vi "rs3_ExtractColor5.vi"(0 "Manual \nWhite Balance":bool, 1 "24bit Color Array":u8[](array[numeric])=array[921600 elements], 2 "AWB SW":bool, 3 "Alpha":dbl, 5 "Red":dbl=2.0, 6 "X offset":dbl, 7 "Color format":enum16{"Monochrome", "RGB internal (RGB)"}(ring), 9 "Green":dbl=1.0, 10 "Depth Y":i32=360, 11 "Blue":dbl=2.0, 12 "RGB  X":i32=640, 13 "Gain":dbl=2.0, 14 "RGB Y":i32=480, 15 "Depth X":i32=480) -> (4 "Norm Mesh Color":T1(array[cluster]))   [LabVIEW 2018, in "libRealSense3.lvlib"]
doc: "Extract the color in a format required for plotting a pointcloud into 3D picture indication"
uses:
  libRealSense3.lvlib
  <vilib>/Analysis/NI_AALBase.lvlib
panel:
  out "New Blue":dbl
  out "New Green":dbl
  out "New Red":dbl
  out "Ratio X":dbl=1.0
  out "Ratio Y":dbl=640.0
  # "RS3 Extract Color for PointCloud"
  # "(C) Intel Corp. 2017,  AGJ"
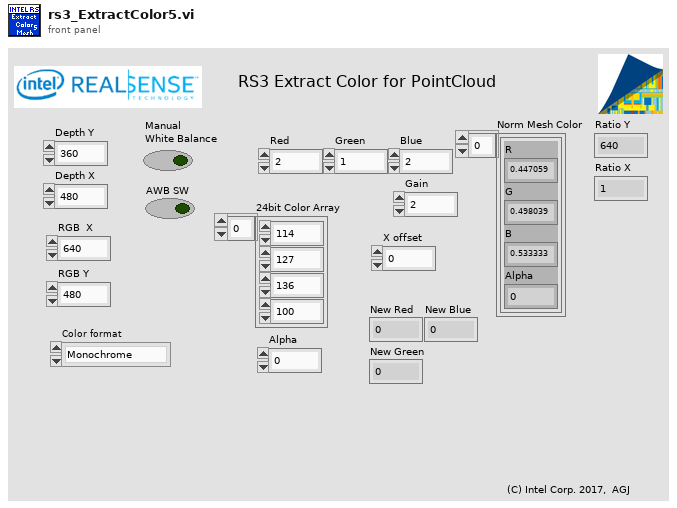
[diagram p1: front panel]
types:
  T1 = cluster{"R":dbl, "G":dbl, "B":dbl, "Alpha":dbl}[]
  T2 = cluster{"upper limit":dbl, "upper limit":dbl, "upper limit":dbl, u8}
  T3 = cluster{"upper limit":dbl, "upper limit":dbl, "upper limit":dbl, "Alpha":dbl}
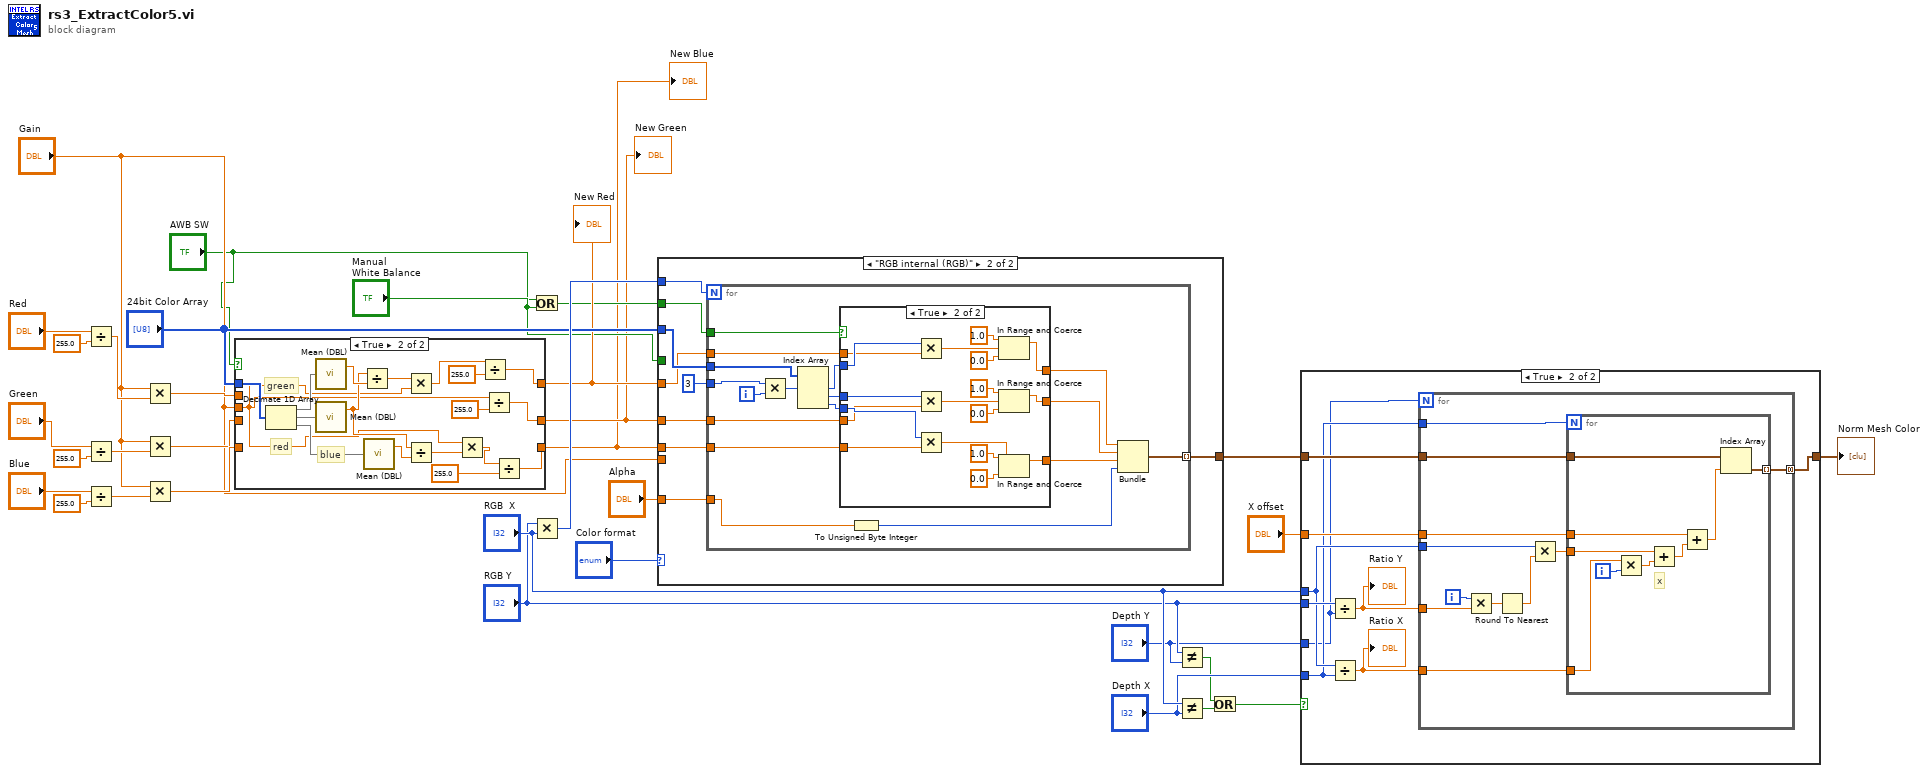
[diagram p0: block diagram]
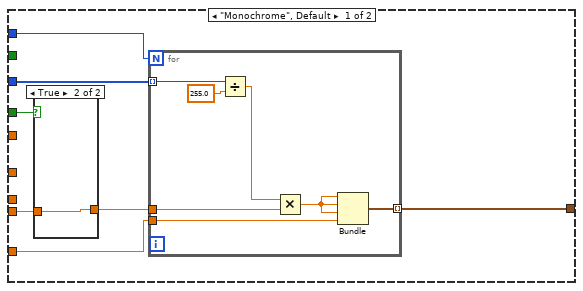
[diagram p3: hidden frame]
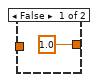
[diagram p4: hidden frame]
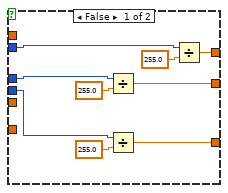
[diagram p5: hidden frame]
diagram:
  n1 = Divide(x="Red", y=255.0 ("upper limit")) -> (x/y=w13:dbl)
  n2 = Divide(x="Green", y=255.0 ("upper limit")) -> (x/y=w12:dbl)
  n3 = Divide(x="Blue", y=255.0 ("upper limit")) -> (x/y=w11:dbl)
  n4 = Multiply(x="Gain", y=w13) -> (x*y=w8:dbl)
  n5 = Multiply(x="Gain", y=w12) -> (x*y=w9:dbl)
  n6 = Multiply(x="Gain", y=w11) -> (x*y=w10:dbl)
  n7 = case shown="True" "AWB SW" {
    tunnel: "24bit Color Array" -> [_ w54]
    tunnel: [w34 w40] -> w14
    tunnel: [w36 w44] -> w2
    tunnel: w9 -> [w36 _]
    tunnel: w10 -> [w35 _]
    tunnel: [w35 w37] -> w1
    tunnel: w8 -> [w34 _]
    tunnel: "Gain" -> [_ w45]
    frame False {
    }
    frame True {
      # "blue"
      # "green"
      # "red"
      n8 = Decimate 1D Array(w54) -> (w53:u8[], w52:u8[], w51:u8[])
      n9 = call <vilib>:"Mean (DBL).vi"("X"=w53) -> ("mean"=w50:dbl)  [unwired: 1 out]
      n10 = call <vilib>:"Mean (DBL).vi"("X"=w52) -> ("mean"=w47:dbl)  [unwired: 1 out]
      n11 = Divide(x=w47, y=w50) -> (x/y=w48:dbl)
      n12 = call <vilib>:"Mean (DBL).vi"("X"=w51) -> ("mean"=w49:dbl)  [unwired: 1 out]
      n13 = Multiply(x=w48, y=w45) -> (x*y=w42:dbl)
      n14 = Divide(x=w47, y=w49) -> (x/y=w46:dbl)
      n15 = Multiply(x=w45, y=w46) -> (x*y=w39:dbl)
      n16 = Divide(x=w42, y=255.0) -> (x/y=w40:dbl)
      n17 = Divide(x=w45, y=255.0) -> (x/y=w44:dbl)
      n18 = Divide(x=w39, y=255.0) -> (x/y=w37:dbl)
    }
  }
  "New Red" <- w14
  "New Green" <- w2
  "New Blue" <- w1
  n19 = Or(x="AWB SW", y="Manual \nWhite Balance") -> (x .or. y?=w4:bool)
  n20 = Multiply(x="RGB Y", y="RGB  X") -> (x*y=w27:i32)
  n21 = case shown="\"RGB internal (RGB)\"" "Color format" {
    tunnel: "24bit Color Array" -> [w60 w79]
    tunnel: w14 -> [_ w77]
    tunnel: w1 -> [_ w76]
    tunnel: w2 -> [_ w75]
    tunnel: "Alpha" -> [w59 w74]
    tunnel: w27 -> [w61 w73]
    tunnel: [w58 w72] -> w26
    tunnel: w4 -> [_ w71]
    tunnel: "Manual \nWhite Balance" -> [w57 _]
    tunnel: "Gain" -> [w56 _]
    frame "Monochrome", Default {
      n22 = case shown="True" w57 {
        tunnel: [1.0 ("Gain") w63] -> w55
        tunnel: w56 -> [_ w63]
        frame False {
        }
        frame True {
        }
      }
      n23 = for {
        N: w61 -> [_]
        tunnel: w60 -> [w68] mode=indexing
        tunnel: [w70] -> w58 mode=indexing
        tunnel: w59 -> [w67]
        tunnel: w55 -> [w65]
        n24 = Divide(x=w68, y=255.0 ("upper limit")) -> (x/y=w66:dbl)
        n25 = Multiply(x=w66, y=w65) -> (x*y=w64:dbl)
        n26 = Bundle(w64, w64, w64, "Alpha"=w67) -> (w70:cluster{dbl, dbl, dbl, "Alpha":dbl})  [unwired: 1 in]
      }
    }
    frame "RGB internal (RGB)" {
      n27 = for {
        N: w73 -> [_]
        tunnel: w79 -> [w94]
        tunnel: 3 ("# of bytes/number") -> [w93]
        tunnel: [w92] -> w72 mode=indexing
        tunnel: w77 -> [w88]
        tunnel: w75 -> [w87]
        tunnel: w76 -> [w86]
        tunnel: w74 -> [w84]
        tunnel: w71 -> [w85]
        i -> [w96]
        n28 = Multiply(x=w93, y=w96) -> (x*y=w95:i32)
        n29 = Index Array(array=w94, index #1=w95) -> (element #1=w91:u8, element #2=w90:u8, element #3=w89:u8)  [unwired: 2 in]
        n30 = case shown="True" w85 {
          tunnel: w91 -> [w104 w123]
          tunnel: w90 -> [w100 w122]
          tunnel: w89 -> [w99 w121]
          tunnel: w88 -> [_ w120]
          tunnel: w87 -> [_ w119]
          tunnel: w86 -> [_ w118]
          tunnel: [w103 w108] -> w80
          tunnel: [w97 w107] -> w81
          tunnel: [w98 w106] -> w82
          frame False {
            n31 = Divide(x=w100, y=255.0 ("upper limit")) -> (x/y=w97:dbl)
            n32 = Divide(x=w99, y=255.0 ("upper limit")) -> (x/y=w98:dbl)
            n33 = Divide(x=w104, y=255.0 ("upper limit")) -> (x/y=w103:dbl)
          }
          frame True {
            n34 = Multiply(x=w123, y=w120) -> (x*y=w117:dbl)
            n35 = Multiply(x=w122, y=w119) -> (x*y=w111:dbl)
            n36 = Multiply(x=w121, y=w118) -> (x*y=w112:dbl)
            n37 = In Range and Coerce(upper limit=1.0, x=w117, lower limit=0.0) -> (coerced(x)=w108:dbl)  [unwired: 1 out]
            n38 = In Range and Coerce(upper limit=1.0, x=w111, lower limit=0.0) -> (coerced(x)=w107:dbl)  [unwired: 1 out]
            n39 = In Range and Coerce(upper limit=1.0, x=w112, lower limit=0.0) -> (coerced(x)=w106:dbl)  [unwired: 1 out]
          }
        }
        n40 = To Unsigned Byte Integer(number=w84) -> (unsigned 8bit integer=w83:u8)
        n41 = Bundle("upper limit"=w80, "upper limit"=w81, "upper limit"=w82, w83) -> (w92:T2)  [unwired: 1 in]
      }
    }
  }
  n42 = Not Equal?(x="RGB Y", y="Depth Y") -> (x != y?=w18:bool)
  n43 = Not Equal?(x="RGB  X", y="Depth X") -> (x != y?=w21:bool)
  n44 = Or(x=w18, y=w21) -> (x .or. y?=w17:bool)
  n45 = case shown="True" w17 {
    tunnel: w26 -> [w124 w133]
    tunnel: [w124 w132] -> w25
    tunnel: "RGB Y" -> [_ w131]
    tunnel: "X offset" -> [_ w130]
    tunnel: "RGB  X" -> [_ w129]
    tunnel: "Depth X" -> [_ w128]
    tunnel: "Depth Y" -> [_ w127]
    frame False {
    }
    frame True {
      n46 = Divide(x=w131, y=w127) -> (x/y=w125:dbl)
      "Ratio Y" <- w125
      n47 = Divide(x=w129, y=w128) -> (x/y=w126:dbl)
      "Ratio X" <- w126
      n48 = for {
        N: w127 -> [_]
        tunnel: w128 -> [w144]
        tunnel: w126 -> [w143]
        tunnel: w125 -> [w140]
        tunnel: w129 -> [w136]
        tunnel: w133 -> [w142]
        tunnel: [w141] -> w132 mode=concatenating
        tunnel: w130 -> [w134]
        i -> [w138]
        n49 = Multiply(x=w138, y=w140) -> (x*y=w139:dbl)
        n50 = Round To Nearest(number=w139) -> (nearest integer value=w137:dbl)
        n51 = Multiply(x=w136, y=w137) -> (x*y=w135:dbl)
        n52 = for {
          N: w144 -> [_]
          tunnel: w143 -> [w152]
          tunnel: w142 -> [w150]
          tunnel: [w149] -> w141 mode=indexing
          tunnel: w135 -> [w148]
          tunnel: w134 -> [w146]
          i -> [w153]
          # "x"
          n53 = Multiply(x=w152, y=w153) -> (x*y=w151:dbl)
          n54 = Add(x=w148, y=w151) -> (x+y=w147:dbl)
          n55 = Add(x=w146, y=w147) -> (x+y=w145:dbl)
          n56 = Index Array(array=w150, index=w145) -> (element=w149:T3)
        }
      }
    }
  }
  "Norm Mesh Color" <- w25
